vi "Find Syncronous Frequency.vi"(9 "DDS clock":dbl=125000000.0 format="%_13p", 10 "DDS modulus":i64=15120 format="0x%x (%d)", 11 "Frequency":dbl format="%#_15p") -> (1 "Points per period":i64, 2 "Frequency word":i64=15120 format="0x%x (%d)", 3 "Actual frequency":dbl format="%_19p", 4 "Remainder":i64)   [LabVIEW 2019]
uses:
  <vilib>/gmath/NI_AAL_MathFunc.lvlib
panel:
  out "Array":i64[](array[numeric])
  out "x+y":i64[](array[numeric])
  out "x*y":i64
  out "x/y":i64
  out "Prime Factors":i64[](array[numeric])
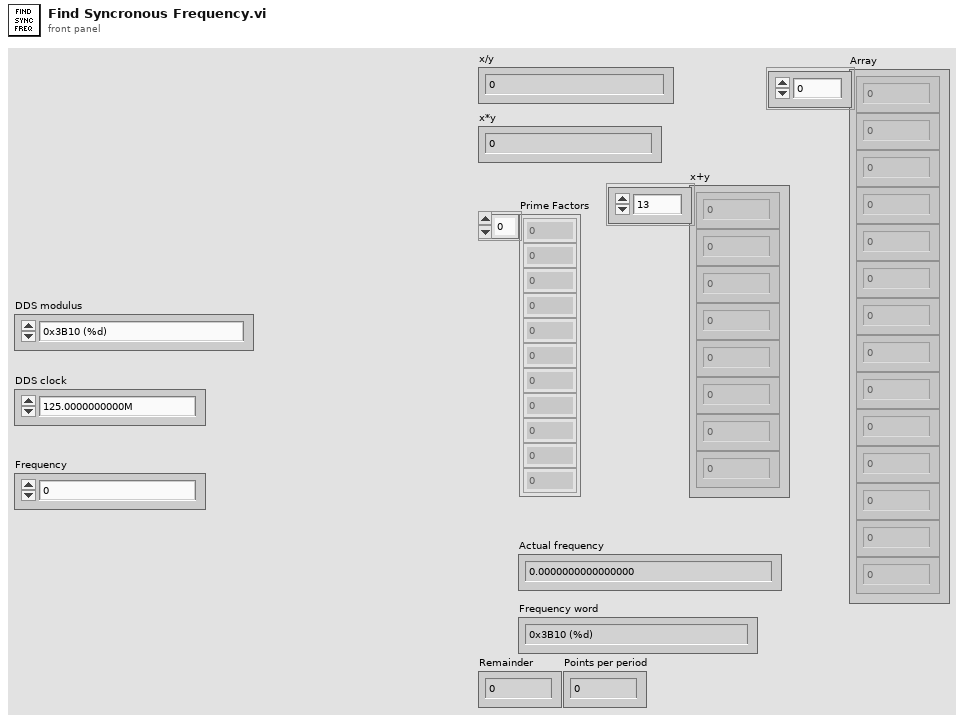
[diagram p1: front panel]
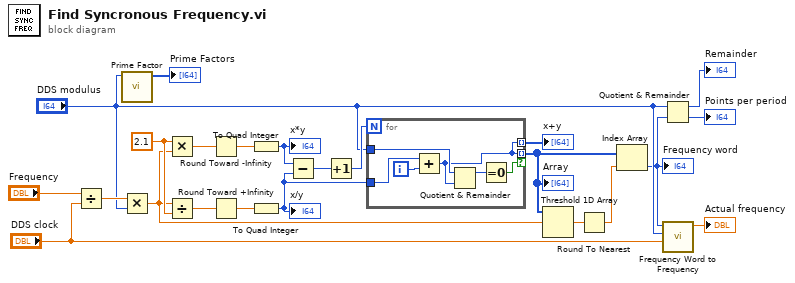
[diagram p0: block diagram]
diagram:
  w22 = 2.1 ("y")
  n1 = Divide(x="Frequency", y="DDS clock") -> (x/y=w20:dbl)
  n2 = call <vilib>:"Prime Factor.vi"("n"="DDS modulus") -> ("Prime Factors"=→"Prime Factors":i64[])  [unwired: 9 in]
  n3 = Multiply(x=w20, y="DDS modulus") -> (x*y=w11:dbl)
  n4 = Multiply(x=w22, y=w11) -> (x*y=w18:dbl)
  n5 = Divide(x=w11, y=w22) -> (x/y=w19:dbl)
  n6 = Round Toward -Infinity(1:w18) -> (0:w17:dbl)
  n7 = Round Toward +Infinity(x=w19) -> (ceil(x): smallest int >= x=w16:dbl)
  n8 = To Quad Integer(1:w17) -> (0:w14:i64)
  "x*y" <- w14
  n9 = To Quad Integer(1:w16) -> (0:w12:i64)
  "x/y" <- w12
  n10 = Subtract(x=w14, y=w12) -> (x-y=w15:i64)
  n11 = Increment(x=w15) -> (x+1=w7:i64)
  n12 = for {
    N: w7 -> [_]
    tunnel: "DDS modulus" -> [w29]
    tunnel: [w24] -> w13 mode=indexing
    tunnel: w12 -> [w28]
    tunnel: [w24] -> w9 mode=indexing if=w25
    i -> [w27]
    n13 = Add(x=w28, y=w27) -> (x+y=w24:i64)
    n14 = Quotient & Remainder(x=w29, y=w24) -> (x-y*floor(x/y)=w26:i64)  [unwired: 1 out]
    n15 = Equal To 0?(x=w26) -> (x = 0?=w25:bool)
  }
  "x+y" <- w13
  "Array" <- w9
  n16 = Threshold 1D Array(2:w11, 3:w9) -> (0:w10:dbl)  [unwired: 1 in]
  n17 = Round To Nearest(number=w10) -> (nearest integer value=w8:dbl)
  n18 = Index Array(array=w9, index=w8) -> (element=w3:i64)
  "Frequency word" <- w3
  n19 = Quotient & Remainder(x="DDS modulus", y=w3) -> (x-y*floor(x/y)=→"Remainder":i64, floor(x/y)=→"Points per period":i64)
  n20 = call "Frequency Word to Frequency .vi"("DDS clock"="DDS clock", "DDS modulus"="DDS modulus", "Frequency word"=w3) -> ("Frequency"=→"Actual frequency":dbl)  [unwired: 8 in]
